vi "Easy Read XML File.vi"(8 "error in (no error)":errorcluster, 9 "LabVIEW Data (Type)":variant, 11 "XML File Path":path) -> (0 "error out":errorcluster, 2 "LabVIEW Data":variant, 3 "XML File Path (duplicate)":path)   [LabVIEW 2013]
doc: "Reads and parses data from an XML file (specified by the <B>XML File Path</B> input), converting it into <B>LabVIEW Data</B>, based on the <B>LabVIEW Data (Type)</B> argument. Use the <B>Variant to Data</B> function to convert the output variant <B>LabVIEW Data</B> to the desired data type."
uses:
  <userlib>/_OpenG.lib/lvdata/lvdata.llb/Type Descriptor Enumeration__ogtk.ctl
panel:
  # "JKI EasyXML Toolkit for LabVIEW\nhttp://jki.net/easyxml\nCopyright (C) 2007-2016, JKI <info@jki.net>\nALL RIGHTS RESERVED"
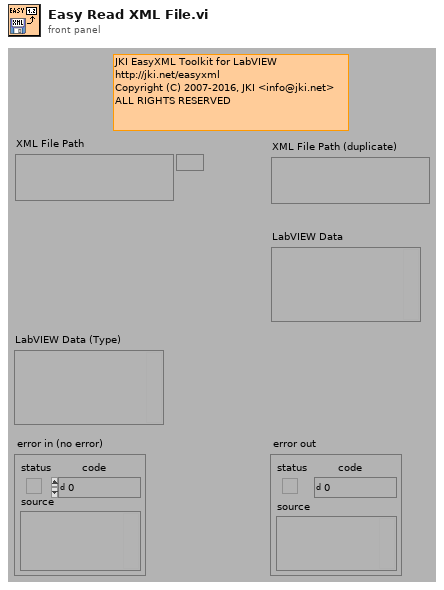
[diagram p1: front panel]
types:
  T1 = typedef "Type Descriptor Enumeration__ogtk.ctl" = enum8{"<Null>", "I8", "I16", "I32", "I64", "U8", "U16", "U32", "U64", "SGL", "DBL", "EXT", "CSG", "CDB", "CXT", "0x0F", "0x10", "0x11", "0x12", "0x13", "0x14", "Enum U8", "Enum U16", "Enum U32", "Enum U64", "SGL PQ", "DBL PQ", "EXT PQ", "CSG PQ", "CDB PQ", "CXT PQ", "0x1F", "0x20", "Boolean", "0x22", "0x23", "0x24", "0x25", "0x26", "0x27", "0x28", "0x29", "0x2A", "0x2B", "0x2C", "0x2D", "0x2E", "0x2F", "String", "0x31", "Path", "Pict", "0x34", "0x35", "0x36", "DAQ", "0x38", "0x39", "0x3A", "0x3B", "0x3C", "0x3D", "0x3E", "0x3F", "Array", "0x41", "0x42", "0x43", "0x44", "0x45", "0x46", "0x47", "0x48", "0x49", "0x4A", "0x4B", "0x4C", "0x4D", "0x4E", "0x4F", "Cluster", "0x51", "0x52", "Variant", "Waveform", "0x55", "0x56", "0x57", "0x58", "0x59", "0x5A", "0x5B", "0x5C", "0x5D", "0x5E", "0x5F", "0x60", "0x61", "0x62", "0x63", "0x64", "0x65", "0x66", "0x67", "0x68", "0x69", "0x6A", "0x6B", "0x6C", "0x6D", "0x6E", "0x6F", "Refnum"}
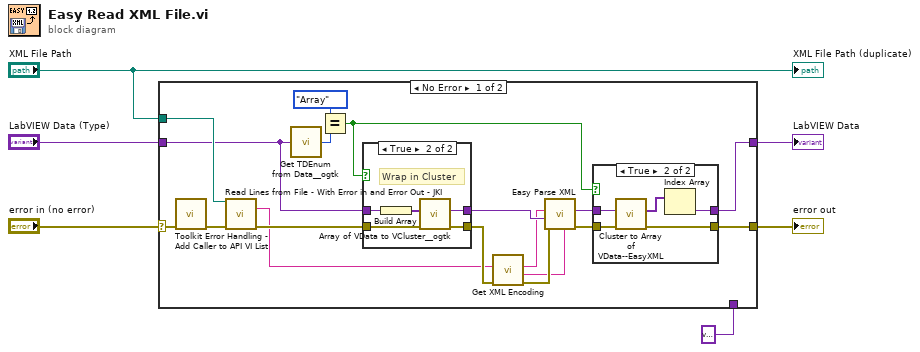
[diagram p0: block diagram]
diagram:
  n1 = case shown="No Error" "error in (no error)" {
    selector: "error in (no error)" -> [w14 w40]
    tunnel: [w17 w40] -> w5
    tunnel: "XML File Path" -> [w24 _]
    tunnel: "LabVIEW Data (Type)" -> [w21 _]
    tunnel: [w15 w39] -> w2
    tunnel: variant ("LabVIEW Data") -> [_ w39]
    frame No Error {
      n2 = call "Toolkit Error Handling - Add Caller to API VI List.vi"("error in"=w14) -> ("error out"=w13:errorcluster)  [unwired: 10 in]
      n3 = call "Read Lines from File - With Error in and Error Out - JKI.vi"("file path (dialog if empty)"=w24, "error in (no error)"=w13) -> ("line string"=w7:string, "error out"=w12:errorcluster)  [unwired: 9 in, 3 out]
      n4 = call <userlib>:"Get TDEnum from Data__ogtk.vi"("Data"=w21) -> ("Type Descriptor Enumeration"=w23:T1)  [unwired: 4 in]
      n5 = Equal?(x=Type_Descriptor_Enumeration__ogtk."Array" ("Type Descriptor Enumeration"), y=w23) -> (x = y?=w16:bool)
      n6 = case shown="True" w16 {
        tunnel: w12 -> [w33 w37]
        tunnel: [w33 w36] -> w11
        tunnel: w21 -> [w32 w35]
        tunnel: [w32 w34] -> w20
        frame False {
        }
        frame True {
          # "Wrap in Cluster"
          n7 = Build Array(w35) -> (w38:variant[])
          n8 = call <userlib>:"Array of VData to VCluster__ogtk.vi"("error in (no error)"=w37, "Array"=w38) -> ("error out"=w36:errorcluster, "VCluster"=w34:variant)  [unwired: 8 in]
        }
      }
      n9 = call "Get XML Encoding.vi"("error in (no error)"=w11, "XML string"=w7) -> ("error out"=w10:errorcluster, "Encoding"=w9:string, "XML string out"=w8:string)  [unwired: 7 in]
      n10 = call "Easy Parse XML.vi"("Encoding (none)"=w9, "error in (no error)"=w10, "LabVIEW Data (Type)"=w20, "XML String"=w8) -> ("error out"=w18:errorcluster, "LabVIEW Data"=w19:variant)  [unwired: 6 in]
      n11 = case shown="True" w16 {
        tunnel: w19 -> [w25 w31]
        tunnel: w18 -> [w26 w30]
        tunnel: [w26 w29] -> w17
        tunnel: [w25 w27] -> w15
        frame False {
        }
        frame True {
          n12 = call "Cluster to Array of VData--EasyXML.vi"("error in (no error)"=w30, "Cluster"=w31) -> ("error out"=w29:errorcluster, "Array of VData"=w28:variant[])  [unwired: 8 in]
          n13 = Index Array(array=w28) -> (element=w27:variant)  [unwired: 1 in]
        }
      }
    }
    frame Error {
    }
  }
  "error out" <- w5
  "LabVIEW Data" <- w2
  "XML File Path (duplicate)" <- "XML File Path"
